vi "Tree_Cluster Tag convert.vi"(11 "Tag":string) -> (0 "Full Element Name":string, 1 "Index":u32, 2 "Tree Nest":string[](array[string]), 3 "Display Name":string, 4 "Is Cluster?":bool, 5 "Unique ID":string)   [LabVIEW 2023]
doc: "Display Name is the last element of the period-delimited tag. Full Element Name is the entire nested tag, except the prepended index (which may also be prepended with \"C\" for cluster). This index makes each tag unique in case a multiple of the same element is on the bundler."
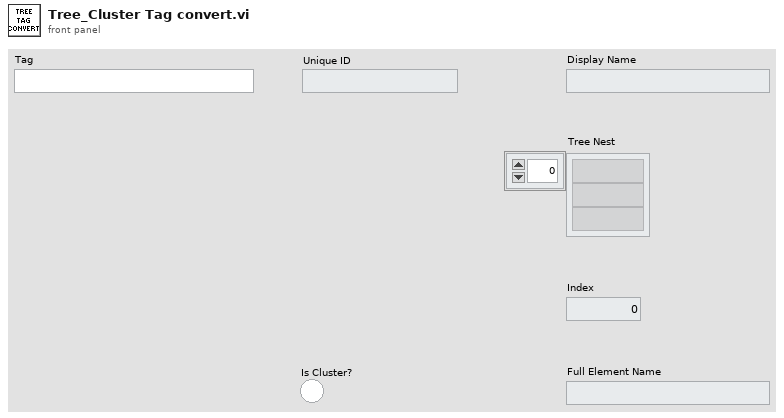
[diagram p1: front panel]
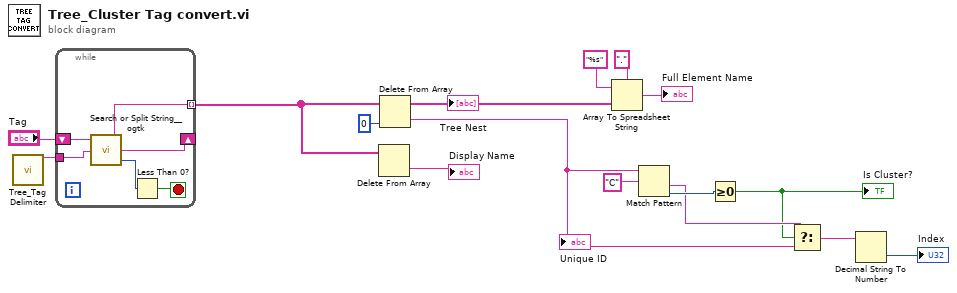
[diagram p0: block diagram]
diagram:
  n1 = call "Tree_Tag Delimiter.vi"() -> ("Tree Tag delimiter"=w10:string)  [unwired: 11 in]
  n2 = while {
    shift-right: [w19] -> _
    shift-left: "Tag" -> [w22]
    tunnel: [w17] -> w6 mode=indexing
    tunnel: w10 -> [w21]
    stop <- w20 stop-if-true
    n3 = call <userlib>:"Search or Split String__ogtk.vi"("search string/char (-)"=w21, "string"=w22) -> ("offset after match"=w18:i32, "substring after match"=w19:string, "substring before match"=w17:string)  [unwired: 1 in]
    n4 = Less Than 0?(x=w18) -> (x < 0?=w20:bool)
  }
  n5 = Delete From Array(array=w6) -> (deleted portion=→"Display Name":string)  [unwired: 2 in, 1 out]
  n6 = Delete From Array(array=w6, index=0) -> (deleted portion=w1:string, array with subset deleted=w5:string[])  [unwired: 1 in]
  "Unique ID" <- w1
  "Tree Nest" <- w5
  n7 = Array To Spreadsheet String(delimiter (Tab)=".", array=w5, 3:"%s" ("delimiter (Tab)")) -> (spreadsheet string=→"Full Element Name":string)
  n8 = Match Pattern(string=w1, regular expression="C") -> (after substring=w13:string, offset past match=w14:i32)  [unwired: 1 in, 2 out]
  n9 = Greater Or Equal To 0?(x=w14) -> (x >= 0?=w12:bool)
  "Is Cluster?" <- w12
  n10 = Select(t=w13, s=w12, f=w1) -> (s? t:f=w11:string)
  n11 = Decimal String To Number(string=w11) -> (number=→"Index":i32)  [unwired: 2 in, 1 out]
